vi "Hatch Panel Intake.vi"   [LabVIEW 2018]
uses:
  <vilib>/Rock Robotics/WPI/Solenoid/WPI_SolenoidChannel.ctl
  <vilib>/Rock Robotics/WPI/Solenoid/WPI_SolenoidValue.ctl
  Hatch Panel Intake Global.vi
  <vilib>/Rock Robotics/WPI/Solenoid/WPI_SolenoidOpenSingle.vi
  Cargo Intake/Cargo Intake Global.vi
  Times/Times Global.vi
  Controllers/Manipulator Controlller/Manipulator Controller Global.vi
  <vilib>/Rock Robotics/WPI/Solenoid/WPI_SolenoidSetEnum.vi
types:
  T1 = typedef "WPI_SolenoidChannel.ctl" = enum8{"Solenoid 0", "Solenoid 1", "Solenoid 2", "Solenoid 3", "Solenoid 4", "Solenoid 5", "Solenoid 6", "Solenoid 7", "Invalid"}
  T2 = enum16{"Full Manual Control", "Manual Control", "Autonomous Control", "Fully Autonomous Control"}
  T3 = typedef "WPI_SolenoidValue.ctl" = enum16{"Off", "On", "Forward", "Reverse"}
  T4 = typedef "WPI_SolenoidDevRef.ctl" = cluster{"DevStatus":errorcluster, "Pneumatics Control Module":u8, "Forward Solenoid Channel":T1, "Reverse Solenoid Channel":T1}
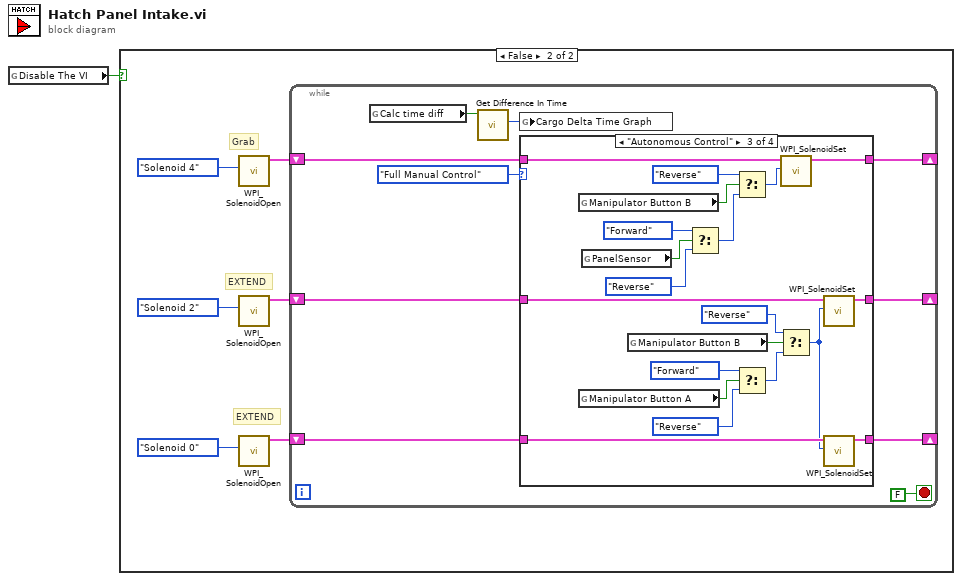
[diagram p0: block diagram]
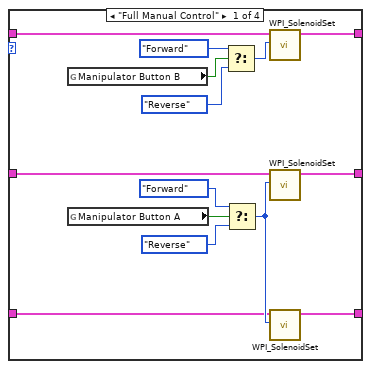
[diagram p3: hidden frame]
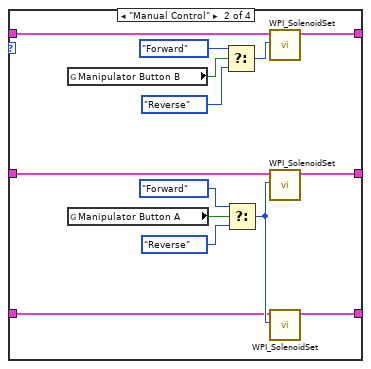
[diagram p4: hidden frame]
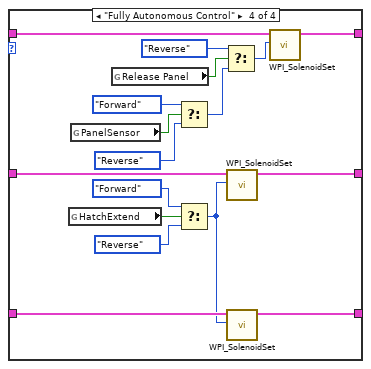
[diagram p5: hidden frame]
diagram:
  n1 = global read "Hatch Panel Intake Global.vi" "Disable The VI"() -> (w1:bool)
  n2 = case shown="False" w1 {
    frame True {
    }
    frame False {
      # "EXTEND"
      # "EXTEND"
      # "Grab"
      n3 = call-poly <vilib>:"WPI_SolenoidOpen.vi"("Solenoid Channel"=WPI_SolenoidChannel."Solenoid 4" ("Forward Solenoid Channel")) -> ("SolenoidDevRef"=w2:T4)  [unwired: 9 in, 1 out]
      n4 = call-poly <vilib>:"WPI_SolenoidOpen.vi"("Solenoid Channel"=WPI_SolenoidChannel."Solenoid 2" ("Forward Solenoid Channel")) -> ("SolenoidDevRef"=w6:T4)  [unwired: 9 in, 1 out]
      n5 = call-poly <vilib>:"WPI_SolenoidOpen.vi"("Solenoid Channel"=WPI_SolenoidChannel."Solenoid 0" ("Forward Solenoid Channel")) -> ("SolenoidDevRef"=w7:T4)  [unwired: 9 in, 1 out]
      n6 = while {
        shift-right: [w12] -> _
        shift-left: w2 -> [w13]
        shift-right: [w11] -> _
        shift-left: w6 -> [w14]
        shift-right: [w10] -> _
        shift-left: w7 -> [w15]
        stop <- FALSE stop-if-true
        n7 = global read "Cargo Intake Global.vi" "Calc time diff"() -> (w9:bool)
        n8 = call "Get Difference In Time.vi"("Calculate Time Difference"=w9) -> ("Delta Time over Time"=w8:u32)  [unwired: 9 in, 1 out]
        n9 = global write "Times Global.vi" "Cargo Delta Time Graph"(w8) -> ()
        n10 = case shown="\"Autonomous Control\"" T2."Full Manual Control" ("Mode") {
          tunnel: w15 -> [w23 w38 w65 w77]
          tunnel: w14 -> [w22 w37 w61 w80]
          tunnel: w13 -> [w21 w36 w63 w81]
          tunnel: [w18 w33 w62 w82] -> w12
          tunnel: [w19 w34 w60 w79] -> w11
          tunnel: [w20 w35 w64 w78] -> w10
          frame "Full Manual Control" {
            n11 = global read "Manipulator Controller Global.vi" "Manipulator Button B"() -> (w25:bool)
            n12 = global read "Manipulator Controller Global.vi" "Manipulator Button A"() -> (w28:bool)
            n13 = Select(t=WPI_SolenoidValue."Forward" ("Value"), s=w25, f=WPI_SolenoidValue."Reverse" ("Value")) -> (s? t:f=w24:T3)
            n14 = Select(t=WPI_SolenoidValue."Forward" ("Value"), s=w28, f=WPI_SolenoidValue."Reverse" ("Value")) -> (s? t:f=w29:T3)
            n15 = call-poly <vilib>:"WPI_SolenoidSet.vi"("Value"=w24, "SolenoidDevRef"=w21) -> ("SolenoidDevRef"=w18:T4)  [unwired: 8 in, 1 out]
            n16 = call-poly <vilib>:"WPI_SolenoidSet.vi"("Value"=w29, "SolenoidDevRef"=w22) -> ("SolenoidDevRef"=w19:T4)  [unwired: 8 in, 1 out]
            n17 = call-poly <vilib>:"WPI_SolenoidSet.vi"("Value"=w29, "SolenoidDevRef"=w23) -> ("SolenoidDevRef"=w20:T4)  [unwired: 8 in, 1 out]
          }
          frame "Manual Control" {
            n18 = global read "Manipulator Controller Global.vi" "Manipulator Button B"() -> (w40:bool)
            n19 = global read "Manipulator Controller Global.vi" "Manipulator Button A"() -> (w43:bool)
            n20 = Select(t=WPI_SolenoidValue."Forward" ("Value"), s=w40, f=WPI_SolenoidValue."Reverse" ("Value")) -> (s? t:f=w39:T3)
            n21 = Select(t=WPI_SolenoidValue."Forward" ("Value"), s=w43, f=WPI_SolenoidValue."Reverse" ("Value")) -> (s? t:f=w44:T3)
            n22 = call-poly <vilib>:"WPI_SolenoidSet.vi"("Value"=w39, "SolenoidDevRef"=w36) -> ("SolenoidDevRef"=w33:T4)  [unwired: 8 in, 1 out]
            n23 = call-poly <vilib>:"WPI_SolenoidSet.vi"("Value"=w44, "SolenoidDevRef"=w37) -> ("SolenoidDevRef"=w34:T4)  [unwired: 8 in, 1 out]
            n24 = call-poly <vilib>:"WPI_SolenoidSet.vi"("Value"=w44, "SolenoidDevRef"=w38) -> ("SolenoidDevRef"=w35:T4)  [unwired: 8 in, 1 out]
          }
          frame "Autonomous Control" {
            n25 = global read "Manipulator Controller Global.vi" "Manipulator Button B"() -> (w59:bool)
            n26 = global read "Manipulator Controller Global.vi" "Manipulator Button A"() -> (w47:bool)
            n27 = global read "Hatch Panel Intake Global.vi" "PanelSensor"() -> (w58:bool)
            n28 = global read "Manipulator Controller Global.vi" "Manipulator Button B"() -> (w51:bool)
            n29 = Select(t=WPI_SolenoidValue."Forward" ("Value"), s=w58, f=WPI_SolenoidValue."Reverse" ("Value")) -> (s? t:f=w57:T3)
            n30 = Select(t=WPI_SolenoidValue."Reverse", s=w59, f=w57) -> (s? t:f=w53:T3)
            n31 = Select(t=WPI_SolenoidValue."Forward" ("Value"), s=w47, f=WPI_SolenoidValue."Reverse" ("Value")) -> (s? t:f=w48:T3)
            n32 = call-poly <vilib>:"WPI_SolenoidSet.vi"("Value"=w53, "SolenoidDevRef"=w63) -> ("SolenoidDevRef"=w62:T4)  [unwired: 8 in, 1 out]
            n33 = Select(t=WPI_SolenoidValue."Reverse" ("Value"), s=w51, f=w48) -> (s? t:f=w46:T3)
            n34 = call-poly <vilib>:"WPI_SolenoidSet.vi"("Value"=w46, "SolenoidDevRef"=w61) -> ("SolenoidDevRef"=w60:T4)  [unwired: 8 in, 1 out]
            n35 = call-poly <vilib>:"WPI_SolenoidSet.vi"("Value"=w46, "SolenoidDevRef"=w65) -> ("SolenoidDevRef"=w64:T4)  [unwired: 8 in, 1 out]
          }
          frame "Fully Autonomous Control" {
            n36 = global read "Hatch Panel Intake Global.vi" "HatchExtend"() -> (w67:bool)
            n37 = global read "Hatch Panel Intake Global.vi" "PanelSensor"() -> (w74:bool)
            n38 = global read "Hatch Panel Intake Global.vi" "Release Panel"() -> (w71:bool)
            n39 = Select(t=WPI_SolenoidValue."Forward" ("Value"), s=w74, f=WPI_SolenoidValue."Reverse" ("Value")) -> (s? t:f=w73:T3)
            n40 = Select(t=WPI_SolenoidValue."Forward" ("Value"), s=w67, f=WPI_SolenoidValue."Reverse" ("Value")) -> (s? t:f=w68:T3)
            n41 = Select(t=WPI_SolenoidValue."Reverse", s=w71, f=w73) -> (s? t:f=w72:T3)
            n42 = call-poly <vilib>:"WPI_SolenoidSet.vi"("Value"=w68, "SolenoidDevRef"=w80) -> ("SolenoidDevRef"=w79:T4)  [unwired: 8 in, 1 out]
            n43 = call-poly <vilib>:"WPI_SolenoidSet.vi"("Value"=w68, "SolenoidDevRef"=w77) -> ("SolenoidDevRef"=w78:T4)  [unwired: 8 in, 1 out]
            n44 = call-poly <vilib>:"WPI_SolenoidSet.vi"("Value"=w72, "SolenoidDevRef"=w81) -> ("SolenoidDevRef"=w82:T4)  [unwired: 8 in, 1 out]
          }
        }
      }
    }
  }
